vi "Teardown.vi"(8 "Error in":errorcluster, 9 "Teardown Location":T1, 10 "Unhandled Msgs":refnum<class "Msg.lvclass">[](array[class]), 11 "Core Actor in":refnum<class "Core Actor.lvclass">) -> (3 "Core Actor out":refnum<class "Core Actor.lvclass">)   [LabVIEW 2025, in "jettl.lvlib" / "Actor.lvlib" / "Core Actor.lvclass"]
uses:
  Core Actor.lvclass
  Teardown Location.ctl
  Msg/Msg.lvclass
  Core Actor.lvclass/Core Actor.ctl
  Actor.lvlib
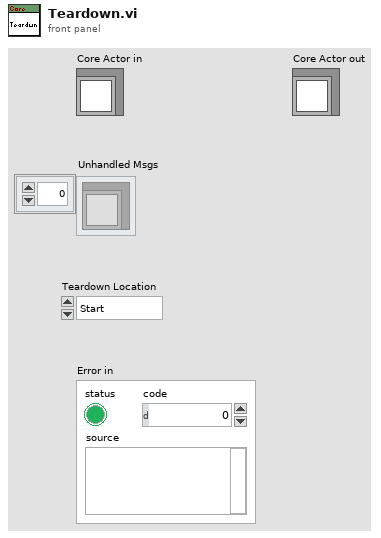
[diagram p1: front panel]
types:
  T1 = typedef "jettl.lvlib/Actor.lvlib/Teardown Location.ctl" = enum16{"Start", "Stop"}
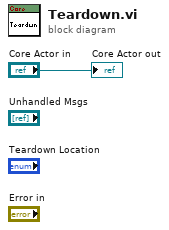
[diagram p0: block diagram]
diagram:
  "Core Actor out" <- "Core Actor in"
